vi "Lakeshore 218 Config GUI.vi"(11 "LS 218 Settings":T1={"Port"="Lakeshore218", "Channel Names"=[], "Ch Enable"=[]}) -> (3 "Settings out":T1={"Port"="Lakeshore218", "Channel Names"=[], "Ch Enable"=[]})   [LabVIEW 2022 SP3, in "Lakeshore 218.lvclass"]
uses:
  Lakeshore 218.lvclass
  Lakeshore 218 cluster Settings.ctl
  Lakeshore 218.lvclass/Lakeshore 218.ctl
panel:
  in  "Cancel Button":bool
  in  "OK Button":bool
  in  "Port":refnum<visa-resource-name>
  in  "Channel Names":cluster{"Enable":bool, "Name":string}[](array[cluster])
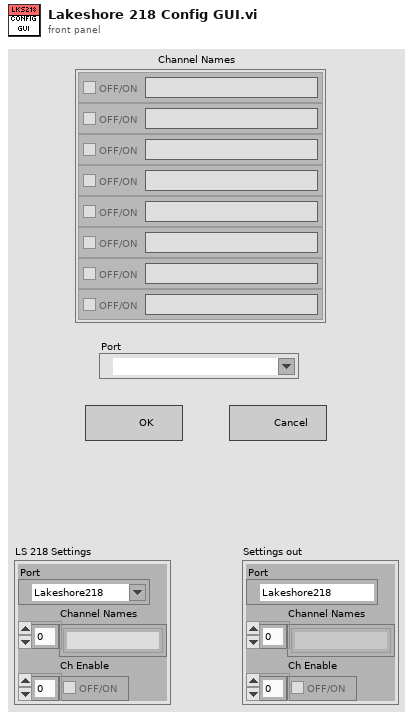
[diagram p1: front panel]
types:
  T1 = typedef "Lakeshore 218.lvclass/Lakeshore 218 cluster Settings.ctl" = cluster{"Port":refnum<visa-resource-name>, "Channel Names":string[], "Ch Enable":bool[]}
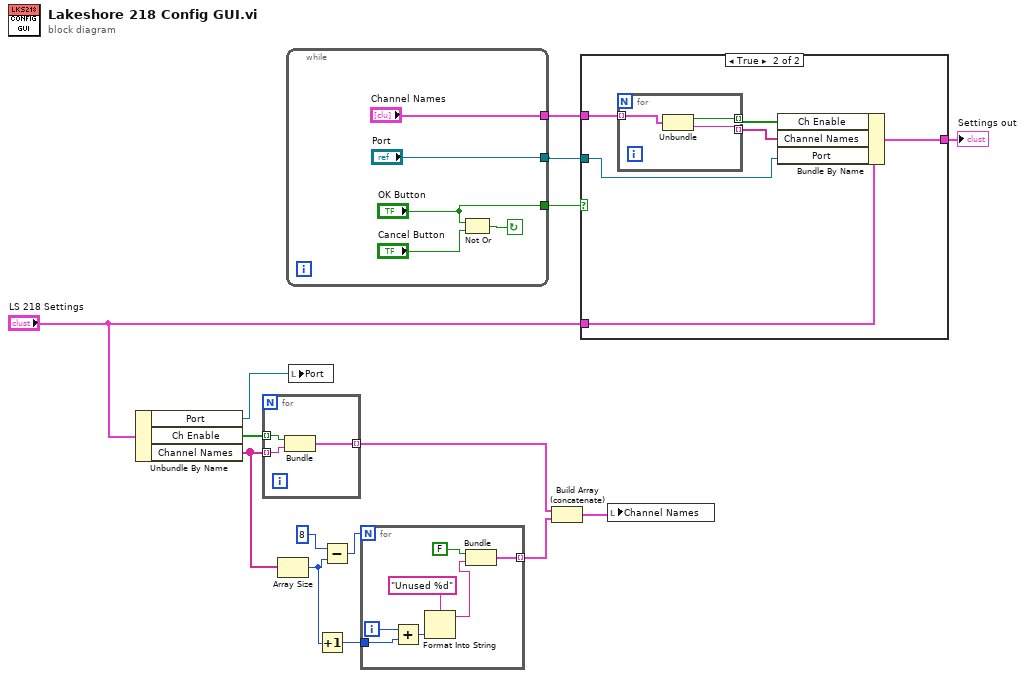
[diagram p0: block diagram]
diagram:
  n1 = Unbundle By Name("LS 218 Settings") -> ("Port"=w8:refnum<visa-resource-name>, "Ch Enable"=w15:bool[], "Channel Names"=w13:string[])
  n2 = for {
    tunnel: w15 -> [w18] mode=indexing
    tunnel: w13 -> [w17] mode=indexing
    tunnel: [w16] -> w10 mode=indexing
    n3 = Bundle("Boolean"=w18, "String"=w17) -> (w16:cluster{"Boolean":bool, "String":string})  [unwired: 1 in]
  }
  n4 = Array Size(array=w13) -> (size(s)=w12:i32)
  n5 = while {
    tunnel: ["Channel Names"] -> w5
    tunnel: ["Port"] -> w4
    tunnel: ["OK Button"] -> w7
    stop <- w22 continue-if-true
    n6 = Not Or(1:"Cancel Button", 2:"OK Button") -> (0:w22:bool)
  }
  n7 = local write "Port"(w8) -> ()
  n8 = Increment(x=w12) -> (x+1=w1:i32)
  n9 = Subtract(x=8, y=w12) -> (x-y=w2:i32)
  n10 = for {
    N: w2 -> [_]
    tunnel: w1 -> [w25]
    tunnel: [w24] -> w11 mode=indexing
    i -> [w30]
    n11 = Add(x=w30, y=w25) -> (x+y=w26:i32)
    n12 = Format Into String(format string="Unused %d", w26) -> (resulting string=w27:string)  [unwired: 2 in, 1 out]
    n13 = Bundle(FALSE, w27) -> (w24:cluster{bool, string})  [unwired: 1 in]
  }
  n14 = Build Array (concatenate)(w10, w11) -> (w9:cluster{"Boolean":bool, "String":string}[])
  n15 = case shown="True" w7 {
    tunnel: "LS 218 Settings" -> [w31 w36]
    tunnel: w5 -> [_ w37]
    tunnel: w4 -> [_ w33]
    tunnel: [w31 w32] -> w3
    frame False {
    }
    frame True {
      n16 = for {
        tunnel: w37 -> [w40] mode=indexing
        tunnel: [w39] -> w35 mode=indexing
        tunnel: [w38] -> w34 mode=indexing
        n17 = Unbundle(w40) -> ("Enable"=w39:bool, "Name"=w38:string)
      }
      n18 = Bundle By Name(cluster=w36, "Ch Enable"=w35, "Channel Names"=w34, "Port"=w33) -> (w32:T1)
    }
  }
  "Settings out" <- w3
  n19 = local write "Channel Names"(w9) -> ()
